vi "LiftCONTROL.vi"(0 "Left Bumper":bool, 1 "Left Trigger":bool, 2 "Manual Control":dbl, 3 "Right Bumper":bool, 4 "Right Trigger":bool) -> ()   [LabVIEW 2020]
uses:
  <vilib>/Rock Robotics/WPI/ThirdParty/Phoenix-LabVIEW/Motor Controller/Controls/CTRE_Phoenix_MotorControl_ControlMode.ctl
  <vilib>/Rock Robotics/WPI/ThirdParty/Phoenix-LabVIEW/Motor Controller/Get/CTRE_Phoenix_MotorController_GetSelectedSensorData.vi
panel:
  out "ecnoder reseted":bool
  in  "Encoder Reset to 200":bool
  in  "Cargo Setpoint 0":i32=200
  in  "Hatch Setpoint 0":i32=200
  in  "Lift Allowed Error":i32=200
  out "hit bottom":bool
  out "Value to Motor":dbl
  in  "Lift DN Speed":dbl=0.5
  in  "Lift UP Speed":dbl=-0.6
  in  "Cargo Setpoint 2":i32=14201
  in  "Cargo Setpoint 1":i32=6821
  in  "Hatch Setpoint 3":i32=14800
  in  "Hatch Setpoint 2":i32=9980
  in  "Hatch Setpoint 1":i32=3079
  out "Encoder SetPoint":i32
  out "Cargo Current Lvl":T1(ring)
  out "Hatch Current Lvl":T2(ring)
  out "Arrived At Setpoint":bool
  in  "Encoder Reset to Zero":bool
  out "Velocity (Raw Sensor Units per 100 ms)":i32
  out "Position (Raw Sensor Units)":i32
  # "Hatch 3 = 14800\nHatch 2 = 9980\nHatch 1 = 3079\nHatch 0 = 200"
  # "Cargo 3 = DNE\nCargo 2 = 14201\nCargo 1 = 6821\nCargo 0 = 200"
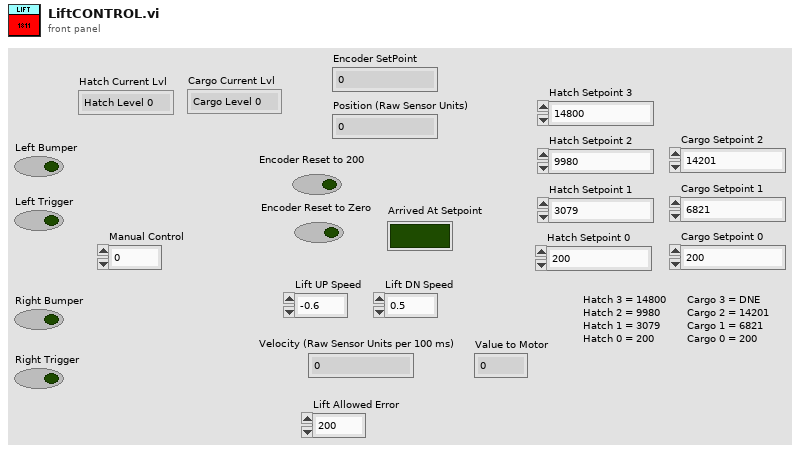
[diagram p1: front panel]
types:
  T1 = enum16{"Cargo Level 0", "Cargo Level 1", "Cargo Level 2"}
  T2 = enum16{"Hatch Level 0", "Hatch Level 1", "Hatch Level 2", "Hatch Level 3"}
  T3 = typedef "CTRE_Phoenix_MotorControl_ControlMode.ctl" = u16
  T4 = typedef "WPI_MotorControlDeviceRef.ctl" = cluster{"DeviceStatus":errorcluster, "Type":T5, "PWM":cluster{"PWM Channel":T6, "DeadBand":T7}, "CAN":cluster{"Device Number":u8, "SetOutput VI Ref":variant, "GetOutput VI Ref":variant, "Enable VI Ref":variant, "Disable VI Ref":variant, "Data":variant}, "Invert":bool, "DIO PWM":cluster{"PWM \"Enable\" Channel":T6, "DIOChannel":T8, "PWM Rate":dbl}}
  T5 = typedef "WPI_MotorControlType.ctl" = enum16{"PWM", "CAN", "DIO PWM"}
  T6 = typedef "FPGA_DIOPWMChannel.ctl" = enum8{"PWM 0", "PWM 1", "PWM 2", "PWM 3", "PWM 4", "PWM 5", "PWM 6", "PWM 7", "PWM 8", "PWM 9", "PWM MXP 0", "PWM MXP 1", "PWM MXP 2", "PWM MXP 3", "PWM MXP 4", "PWM MXP 5", "PWM MXP 6", "PWM MXP 7", "PWM MXP 8", "PWM MXP 9", "Invalid"}
  T7 = typedef "WPI_PWMDeadband.ctl" = cluster{"Name":string, "maxPositivePwm":i32, "minPositivePwm":i32, "centerPwm":i32, "maxNegativePwm":i32, "minNegativePwm":i32, "angularRange":u16}
  T8 = typedef "FPGA_DIOChannel.ctl" = enum8{"DIO 0", "DIO 1", "DIO 2", "DIO 3", "DIO 4", "DIO 5", "DIO 6", "DIO 7", "DIO 8", "DIO 9", "DIO MXP 0", "DIO MXP 1", "DIO MXP 2", "DIO MXP 3", "DIO MXP 4", "DIO MXP 5", "DIO MXP 6", "DIO MXP 7", "DIO MXP 8", "DIO MXP 9", "DIO MXP 10", "DIO MXP 11", "DIO MXP 12", "DIO MXP 13", "DIO MXP 14", "DIO MXP 15", "SPI Port CS1", "SPI Port CS2", "SPI Port CS3", "SPI Port MISO", "SPI Port MOSI", "Invalid"}
  T9 = typedef "WPI_SwitchDevRef.ctl" = cluster{"DevStatus":errorcluster, "DIO Channel":T8, "CntIndex":T10, "Normally Closed":bool}
  T10 = typedef "FPGA_CounterCtrSystemIndex.ctl" = enum8{"Ctr 0", "Ctr 1", "Ctr 2", "Ctr 3", "Ctr 4", "Ctr 5", "Ctr 6", "Ctr 7", "Invalid"}
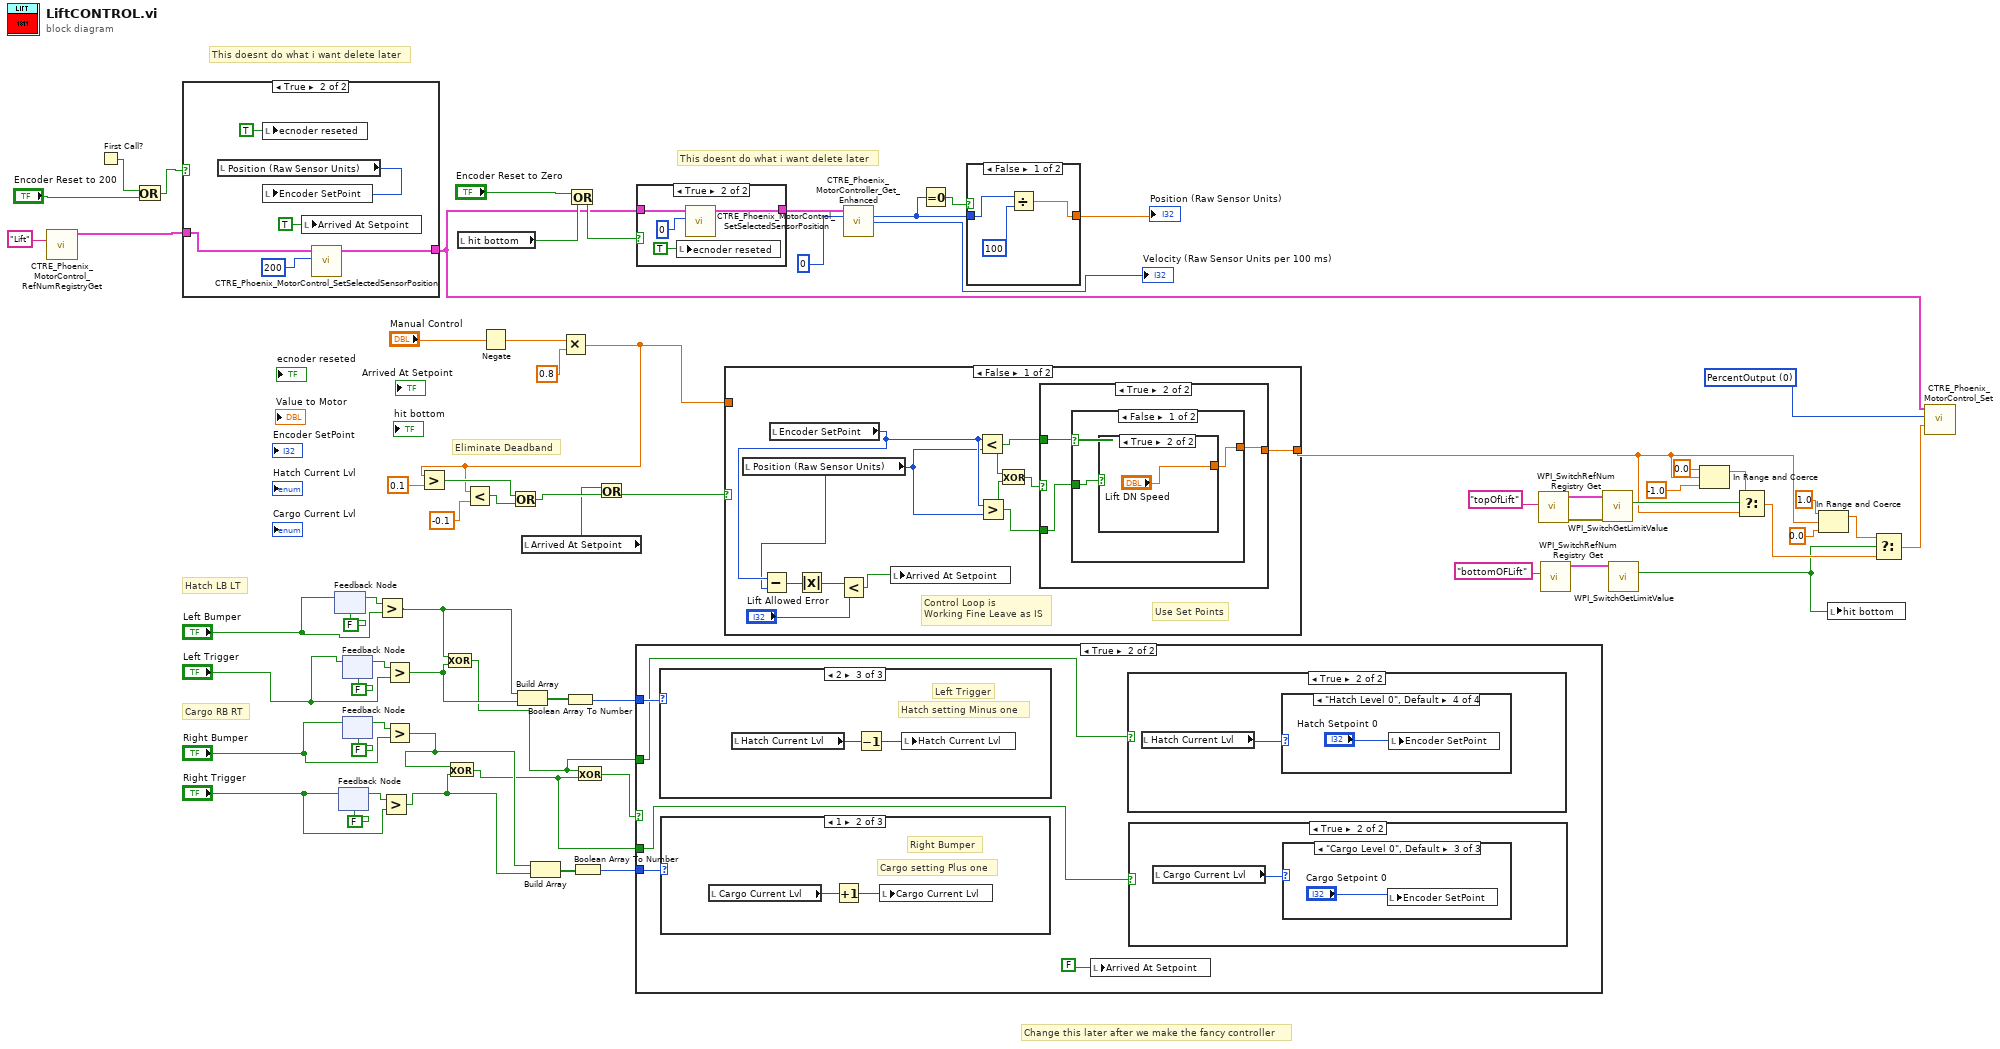
[diagram p0: block diagram]
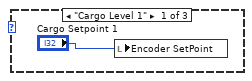
[diagram p5: hidden frame]
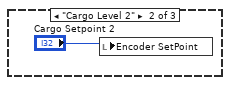
[diagram p6: hidden frame]
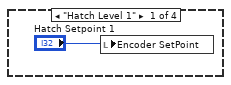
[diagram p8: hidden frame]
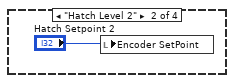
[diagram p9: hidden frame]
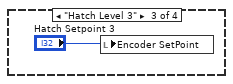
[diagram p10: hidden frame]
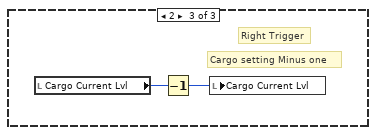
[diagram p12: hidden frame]
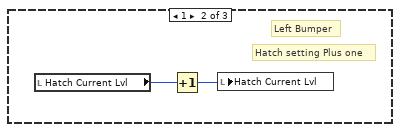
[diagram p14: hidden frame]
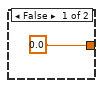
[diagram p15: hidden frame]
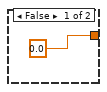
[diagram p16: hidden frame]
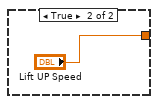
[diagram p17: hidden frame]
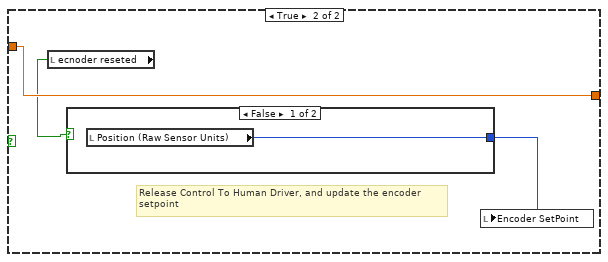
[diagram p18: hidden frame]
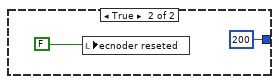
[diagram p19: hidden frame]
diagram:
  w66 = T3 0 items=["PercentOutput"=0, "Position"=1, "Velocity"=2, "Current"=3, "Follower"=5, "MotionProfile"=6, "MotionMagic"=7, "MotionProfileArc"=10, "Disabled"=15] ("Control Mode")
  # "This doesnt do what i want delete later"
  # "This doesnt do what i want delete later"
  # "Change this later after we make the fancy controller"
  # "Eliminate Deadband"
  # "Cargo RB RT"
  # "Hatch LB LT"
  n1 = call <vilib>:"CTRE_Phoenix_MotorControl_RefNumRegistryGet.vi"("refnum name"="Lift") -> ("PhoenixMotorControlDevRef"=w7:T4)  [unwired: 9 in, 1 out]
  n2 = First Call?() -> (First Call?: T/F=w3:bool)
  n3 = Or(x=w3, y="Encoder Reset to 200") -> (x .or. y?=w2:bool)
  n4 = case shown="True" w2 {
    tunnel: w7 -> [w67 w71]
    tunnel: [w67 w69] -> w6
    frame False {
    }
    frame True {
      n5 = local read "Position (Raw Sensor Units)"() -> (w73:i32)
      n6 = local write "ecnoder reseted"(TRUE ("ecnoder reseted")) -> ()
      n7 = local write "Encoder SetPoint"(w73) -> ()
      n8 = local write "Arrived At Setpoint"(TRUE ("Arrived At Setpoint")) -> ()
      n9 = call <vilib>:"CTRE_Phoenix_MotorControl_SetSelectedSensorPosition.vi"("New Sensor Position"=200, "PhoenixMotorControlDevRef"=w71) -> ("PhoenixMotorControlDevRef"=w69:T4)  [unwired: 8 in, 1 out]
    }
  }
  n10 = feedback-in #1("Left Bumper") -> ()
  n11 = feedback #1(FALSE) -> (w23:bool)
  n12 = feedback #2(FALSE) -> (w12:bool)
  n13 = feedback-in #2("Right Trigger") -> ()
  n14 = feedback #3(FALSE) -> (w20:bool)
  n15 = feedback-in #3("Left Trigger") -> ()
  n16 = feedback #4(FALSE) -> (w15:bool)
  n17 = feedback-in #4("Right Bumper") -> ()
  n18 = Greater?(x=w23, y="Left Bumper") -> (0:w21:bool)
  n19 = Greater?(x=w12, y="Right Trigger") -> (0:w9:bool)
  n20 = Greater?(x=w20, y="Left Trigger") -> (0:w18:bool)
  n21 = Greater?(x=w15, y="Right Bumper") -> (0:w13:bool)
  n22 = Exclusive Or(1:w18, 2:w21) -> (0:w5:bool)
  n23 = Exclusive Or(1:w9, 2:w13) -> (0:w4:bool)
  n24 = local read "hit bottom"() -> (w27:bool)
  n25 = Negate(x="Manual Control") -> (-x=w64:dbl)
  n26 = Build Array(w21, w18) -> (w50:bool[])
  n27 = local read "Arrived At Setpoint"() -> (w46:bool)
  n28 = Build Array(w13, w9) -> (w45:bool[])
  n29 = Multiply(x=w64, y=0.8) -> (x*y=w28:dbl)
  n30 = Greater?(x=w28, y=0.1) -> (0:w54:bool)
  n31 = Less?(x=w28, y=-0.1) -> (x < y?=w55:bool)
  n32 = Or(x=w54, y=w55) -> (x .or. y?=w53:bool)
  n33 = Boolean Array To Number(Boolean array=w50) -> (number=w49:u32)
  n34 = Or(x="Encoder Reset to Zero", y=w27) -> (x .or. y?=w48:bool)
  n35 = Boolean Array To Number(Boolean array=w45) -> (number=w44:u32)
  n36 = Exclusive Or(1:w4, 2:w5) -> (0:w43:bool)
  n37 = Or(x=w46, y=w53) -> (x .or. y?=w47:bool)
  n38 = case shown="True" w43 {
    tunnel: w49 -> [_ w78]
    tunnel: w44 -> [_ w77]
    tunnel: w5 -> [_ w75]
    tunnel: w4 -> [_ w74]
    frame False {
    }
    frame True {
      n39 = case shown="2" w78 {
        frame 0, Default {
        }
        frame 1 {
          # "Hatch setting Plus one"
          # "Left Bumper"
          n40 = local read "Hatch Current Lvl"() -> (w93:T2)
          n41 = Increment(x=w93) -> (x+1=w92:T2)
          n42 = local write "Hatch Current Lvl"(w92) -> ()
        }
        frame 2 {
          # "Hatch setting Minus one"
          # "Left Trigger"
          n43 = local read "Hatch Current Lvl"() -> (w95:T2)
          n44 = Decrement(x=w95) -> (x-1=w94:T2)
          n45 = local write "Hatch Current Lvl"(w94) -> ()
        }
      }
      n46 = case shown="1" w77 {
        frame 0, Default {
        }
        frame 1 {
          # "Cargo setting Plus one"
          # "Right Bumper"
          n47 = local read "Cargo Current Lvl"() -> (w89:T1)
          n48 = Increment(x=w89) -> (x+1=w88:T1)
          n49 = local write "Cargo Current Lvl"(w88) -> ()
        }
        frame 2 {
          # "Cargo setting Minus one"
          # "Right Trigger"
          n50 = local read "Cargo Current Lvl"() -> (w91:T1)
          n51 = Decrement(x=w91) -> (x-1=w90:T1)
          n52 = local write "Cargo Current Lvl"(w90) -> ()
        }
      }
      n53 = local write "Arrived At Setpoint"(FALSE ("Arrived At Setpoint")) -> ()
      n54 = case shown="True" w75 {
        frame False {
        }
        frame True {
          n55 = local read "Hatch Current Lvl"() -> (w83:T2)
          n56 = case shown="\"Hatch Level 0\", Default" w83 {
            frame "Hatch Level 1" {
              n57 = local write "Encoder SetPoint"("Hatch Setpoint 1") -> ()
            }
            frame "Hatch Level 2" {
              n58 = local write "Encoder SetPoint"("Hatch Setpoint 2") -> ()
            }
            frame "Hatch Level 3" {
              n59 = local write "Encoder SetPoint"("Hatch Setpoint 3") -> ()
            }
            frame "Hatch Level 0", Default {
              n60 = local write "Encoder SetPoint"("Hatch Setpoint 0") -> ()
            }
          }
        }
      }
      n61 = case shown="True" w74 {
        frame False {
        }
        frame True {
          n62 = local read "Cargo Current Lvl"() -> (w79:T1)
          n63 = case shown="\"Cargo Level 0\", Default" w79 {
            frame "Cargo Level 1" {
              n64 = local write "Encoder SetPoint"("Cargo Setpoint 1") -> ()
            }
            frame "Cargo Level 2" {
              n65 = local write "Encoder SetPoint"("Cargo Setpoint 2") -> ()
            }
            frame "Cargo Level 0", Default {
              n66 = local write "Encoder SetPoint"("Cargo Setpoint 0") -> ()
            }
          }
        }
      }
    }
  }
  n67 = case shown="True" w48 {
    tunnel: w6 -> [w96 w100]
    tunnel: [w96 w99] -> w60
    frame False {
    }
    frame True {
      n68 = local write "ecnoder reseted"(TRUE ("ecnoder reseted")) -> ()
      n69 = call <vilib>:"CTRE_Phoenix_MotorControl_SetSelectedSensorPosition.vi"("New Sensor Position"=0, "PhoenixMotorControlDevRef"=w100) -> ("PhoenixMotorControlDevRef"=w99:T4)  [unwired: 8 in, 1 out]
    }
  }
  n70 = case shown="False" w47 {
    tunnel: w28 -> [_ w122]
    tunnel: [w108 w122] -> w30
    frame False {
      # "Control Loop is \nWorking Fine Leave as IS"
      # "Use Set Points"
      n71 = local read "Position (Raw Sensor Units)"() -> (w105:i32)
      n72 = local read "Encoder SetPoint"() -> (w106:i32)
      n73 = Subtract(x=w106, y=w105) -> (x-y=w104:i32)
      n74 = Absolute Value(x=w104) -> (abs(x)=w102:i32)
      n75 = Less?(x=w102, y="Lift Allowed Error") -> (x < y?=w101:bool)
      n76 = local write "Arrived At Setpoint"(w101) -> ()
      n77 = Less?(x=w106, y=w105) -> (x < y?=w110:bool)
      n78 = Greater?(x=w106, y=w105) -> (0:w109:bool)
      n79 = Exclusive Or(1:w109, 2:w110) -> (0:w107:bool)
      n80 = case shown="True" w107 {
        tunnel: w110 -> [_ w114]
        tunnel: w109 -> [_ w112]
        tunnel: [0.0 w113] -> w108
        frame False {
        }
        frame True {
          n81 = case shown="False" w114 {
            tunnel: [w115 "Lift UP Speed"] -> w113
            tunnel: w112 -> [w116 _]
            frame False {
              n82 = case shown="True" w116 {
                tunnel: [0.0 "Lift DN Speed"] -> w115
                frame False {
                }
                frame True {
                }
              }
            }
            frame True {
            }
          }
        }
      }
    }
    frame True {
      # "Release Control To Human Driver, and update the encoder\nsetpoint"
      n83 = local read "ecnoder reseted"() -> (w120:bool)
      n84 = case shown="False" w120 {
        tunnel: [w123 200 ("Position (Raw Sensor Units)")] -> w121
        frame False {
          n85 = local read "Position (Raw Sensor Units)"() -> (w123:i32)
        }
        frame True {
          n86 = local write "ecnoder reseted"(FALSE) -> ()
        }
      }
      n87 = local write "Encoder SetPoint"(w121) -> ()
    }
  }
  n88 = call-poly <vilib>:"CTRE_Phoenix_MotorController_Get_Enhanced.vi"("PhoenixMotorControlDevRef"=w60, "pidLoopIdx"=u32 0) -> ("Position (Raw Sensor Units)"=w59:i32, "Velocity (Raw Sensor Units per 100 ms)"=→"Velocity (Raw Sensor Units per 100 ms)":i32)  [unwired: 10 in, 2 out]
  n89 = Equal To 0?(x=w59) -> (x = 0?=w58:bool)
  n90 = case shown="False" w58 {
    tunnel: w59 -> [w128 w129]
    tunnel: [w126 w129] -> w51
    frame False {
      n91 = Divide(x=w128, y=100) -> (x/y=w126:dbl)
    }
    frame True {
    }
  }
  "Position (Raw Sensor Units)" <- w51
  n92 = call <vilib>:"WPI_SwitchRefNum Registry Get.vi"("refnum name"="topOfLift") -> ("error out"=w41:errorcluster, "SwitchDevRef"=w40:T9)  [unwired: 9 in]
  n93 = call <vilib>:"WPI_SwitchRefNum Registry Get.vi"("refnum name"="bottomOFLift") -> ("SwitchDevRef"=w42:T9)  [unwired: 9 in, 1 out]
  n94 = call <vilib>:"WPI_SwitchGetLimitValue.vi"("error in (no error)"=w41, "SwitchDevRef"=w40) -> ("Switch Pressed"=w37:bool)  [unwired: 7 in, 2 out]
  n95 = call <vilib>:"WPI_SwitchGetLimitValue.vi"("SwitchDevRef"=w42) -> ("Switch Pressed"=w25:bool)  [unwired: 8 in, 2 out]
  n96 = In Range and Coerce(upper limit=0.0, x=w30, lower limit=-1.0) -> (coerced(x)=w36:dbl)  [unwired: 1 out]
  n97 = Select(t=w36, s=w37, f=w30) -> (s? t:f=w31:dbl)
  n98 = In Range and Coerce(upper limit=1.0, x=w30, lower limit=0.0) -> (coerced(x)=w33:dbl)  [unwired: 1 out]
  n99 = local write "hit bottom"(w25) -> ()
  n100 = Select(t=w33, s=w25, f=w31) -> (s? t:f=w29:dbl)
  n101 = call <vilib>:"CTRE_Phoenix_MotorControl_Set.vi"("Output"=w29, "Control Mode"=w66, "PhoenixMotorControlDevRef"=w6) -> ()  [unwired: 7 in, 2 out]
